vi "Polynomial GCD Pair.vi"   [LabVIEW 2018, in "NI_AALPro.lvlib"]
uses:
  NI_AALPro.lvlib
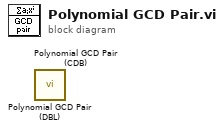
[diagram p0: block diagram]
diagram:
  n1 = call "Polynomial GCD Pair (DBL).vi"() -> ()  [unwired: 8 in, 4 out]
  n2 = call "Polynomial GCD Pair (CDB).vi"() -> ()  [unwired: 8 in, 4 out]
